vi "DepthSense Connect Callback 2.vi"(4 "User Parameter":variant, 6 "Control Ref":refnum<k24>, 7 "Event Common Data":T1) -> ()   [LabVIEW 2011]
uses:
  C:/Users/Behavior Room/Desktop/Kinect Mouse/DepthSense/FunctionPointerProxy/FunctionPointerProxy/bin/Release/FunctionPointerProxy.dll
  FunctionPointerProxy/FunctionPointerProxy/bin/Release/FunctionPointerProxy.dll
  DepthSense Global Status.vi
  <userlib>/libOptrima-2-3/libOptrima-2-3.lvlib
panel:
  out "error out":errorcluster
  out "camera version":string
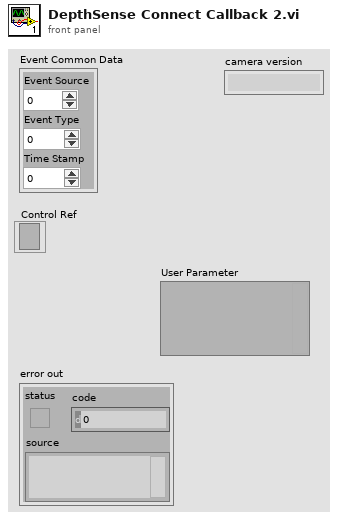
[diagram p1: front panel]
types:
  T1 = cluster{"Event Source":i32, "Event Type":u32, "Time Stamp":u32}
  T2 = typedef "DepthSense State.ctl" = cluster{"Camera Version":string, "Image Height":i32, "Image Width":i32, "Minimum Framerate":i32, "Maximum Framerate":i32, "Framerate":i32, "Close Mode":bool, "Denoising":bool, "Leakage Algorithm":bool, "Anti-Aliasing":bool, "Camera Status":i32, "API Version":string, "Light Intensity":i32}
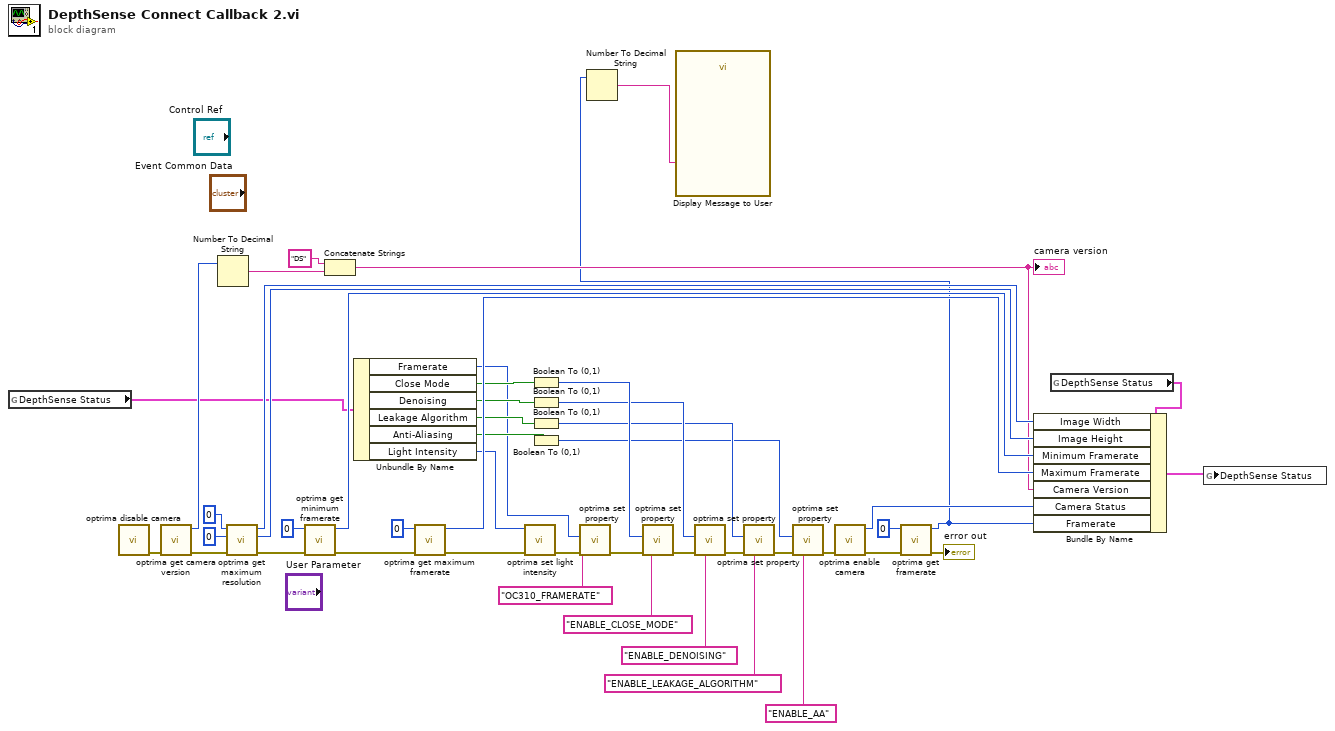
[diagram p0: block diagram]
diagram:
  n1 = global read "DepthSense Global Status.vi" "DepthSense Status"() -> (w3:T2)
  n2 = call <userlib>:"optrima disable camera.vi"() -> ("error out"=w47:errorcluster)  [unwired: 10 in, 1 out]
  n3 = call <userlib>:"optrima get camera version.vi"("error in (no error)"=w47) -> ("error out"=w35:errorcluster, "version out"=w46:u32)  [unwired: 8 in, 1 out]
  n4 = Number To Decimal String(number=w46) -> (decimal integer string=w45:string)  [unwired: 1 in]
  n5 = call <userlib>:"optrima get maximum resolution.vi"("error in (no error)"=w35, "rows"=u32 0, "columns"=u32 0) -> ("error out"=w41:errorcluster, "rows out"=w24:u32, "columns out"=w25:u32)  [unwired: 5 in, 1 out]
  n6 = call <userlib>:"optrima get minimum framerate.vi"("error in (no error)"=w41, "min_framerate"=u32 0) -> ("error out"=w39:errorcluster, "min_framerate out"=w23:u32)  [unwired: 7 in, 1 out]
  n7 = Concatenate Strings("DS" ("string"), w45) -> (w21:string)
  "camera version" <- w21
  n8 = Unbundle By Name(w3) -> ("Framerate"=w6:i32, "Close Mode"=w20:bool, "Denoising"=w19:bool, "Leakage Algorithm"=w18:bool, "Anti-Aliasing"=w17:bool, "Light Intensity"=w8:i32)
  n9 = call <userlib>:"optrima get maximum framerate.vi"("error in (no error)"=w39, "max_framerate"=u32 0) -> ("error out"=w12:errorcluster, "max_framerate out"=w22:u32)  [unwired: 7 in, 1 out]
  n10 = call <userlib>:"optrima set light intensity.vi"("error in (no error)"=w12, "intensity_percentage"=w8) -> ("error out"=w37:errorcluster)  [unwired: 8 in, 1 out]
  n11 = Boolean To (0,1)(Boolean=w20) -> (0, 1=w16:i16)
  n12 = Boolean To (0,1)(Boolean=w19) -> (0, 1=w15:i16)
  n13 = Boolean To (0,1)(Boolean=w18) -> (0, 1=w14:i16)
  n14 = Boolean To (0,1)(Boolean=w17) -> (0, 1=w13:i16)
  n15 = call <userlib>:"optrima set property.vi"("error in (no error)"=w37, "value"=w6, "name"="OC310_FRAMERATE") -> ("error out"=w34:errorcluster)  [unwired: 7 in, 1 out]
  n16 = call <userlib>:"optrima set property.vi"("error in (no error)"=w34, "value"=w16, "name"="ENABLE_CLOSE_MODE") -> ("error out"=w30:errorcluster)  [unwired: 7 in, 1 out]
  n17 = call <userlib>:"optrima set property.vi"("error in (no error)"=w30, "value"=w15, "name"="ENABLE_DENOISING") -> ("error out"=w29:errorcluster)  [unwired: 7 in, 1 out]
  n18 = call <userlib>:"optrima set property.vi"("error in (no error)"=w29, "value"=w14, "name"="ENABLE_LEAKAGE_ALGORITHM") -> ("error out"=w28:errorcluster)  [unwired: 7 in, 1 out]
  n19 = call <userlib>:"optrima set property.vi"("error in (no error)"=w28, "value"=w13, "name"="ENABLE_AA") -> ("error out"=w33:errorcluster)  [unwired: 7 in, 1 out]
  n20 = call <userlib>:"optrima enable camera.vi"("error in (no error)"=w33) -> ("error out"=w10:errorcluster, "function return"=w5:u32)  [unwired: 9 in]
  n21 = call <userlib>:"optrima get framerate.vi"("error in (no error)"=w10, "framerate"=u32 0) -> ("error out"=→"error out":errorcluster, "framerate out"=w4:u32)  [unwired: 7 in, 1 out]
  n22 = Number To Decimal String(number=w4) -> (decimal integer string=w7:string)  [unwired: 1 in]
  n23 = call "Display Message to User"("Message"=w7) -> ()  [unwired: 9 in, 2 out]
  n24 = global read "DepthSense Global Status.vi" "DepthSense Status"() -> (w1:T2)
  n25 = Bundle By Name(cluster=w1, "Image Width"=w25, "Image Height"=w24, "Minimum Framerate"=w23, "Maximum Framerate"=w22, "Camera Version"=w21, "Camera Status"=w5, "Framerate"=w4) -> (w2:T2)
  n26 = global write "DepthSense Global Status.vi" "DepthSense Status"(w2) -> ()
